vi "TestMatrix.vi"() -> ()   [LabVIEW 2022 SP3]
uses:
  <vilib>/Analysis/2dsp.llb/2D Convolution (DBL).vi
  <vilib>/Analysis/NI_AALPro.lvlib
panel:
  out "Intensity Graph 2":dbl[][](graph)
  out "Power":dbl
  out "Time (s)":dbl
  in  "stop":bool
  out "Intensity Graph":dbl[][](graph)
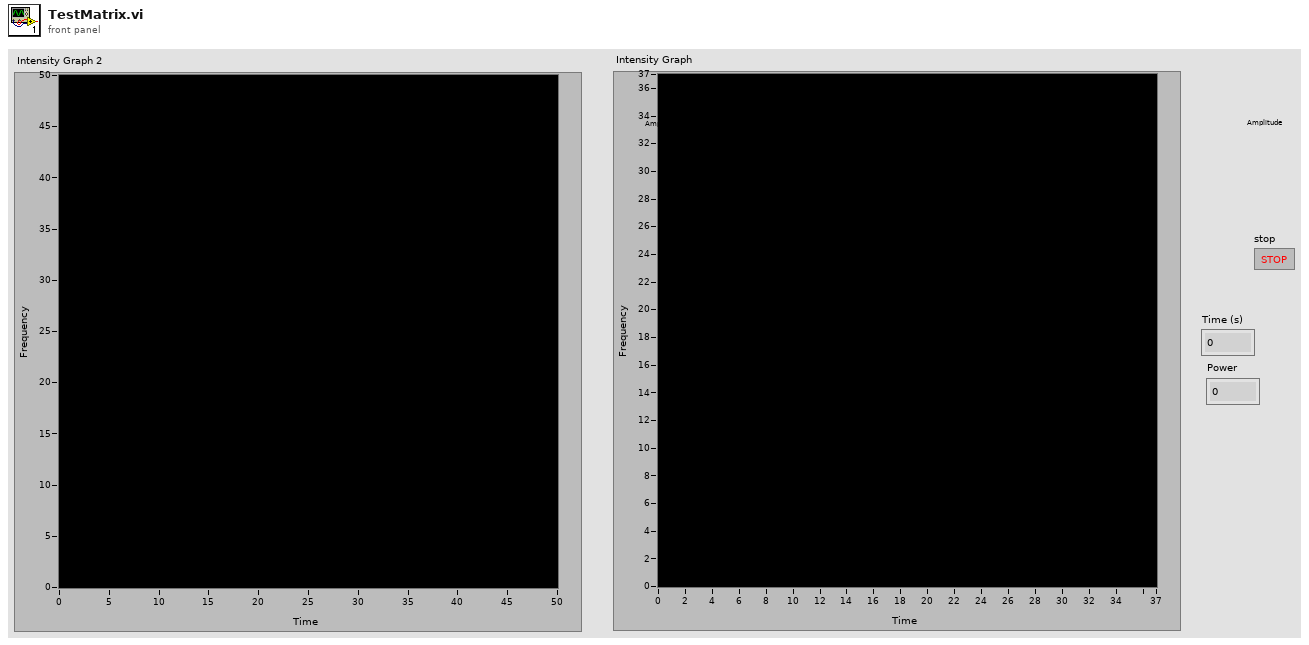
[diagram p1: front panel]
types:
  T1 = enum16{"open", "replace", "create", "open or create", "replace or create", "replace or create with confirmation"}
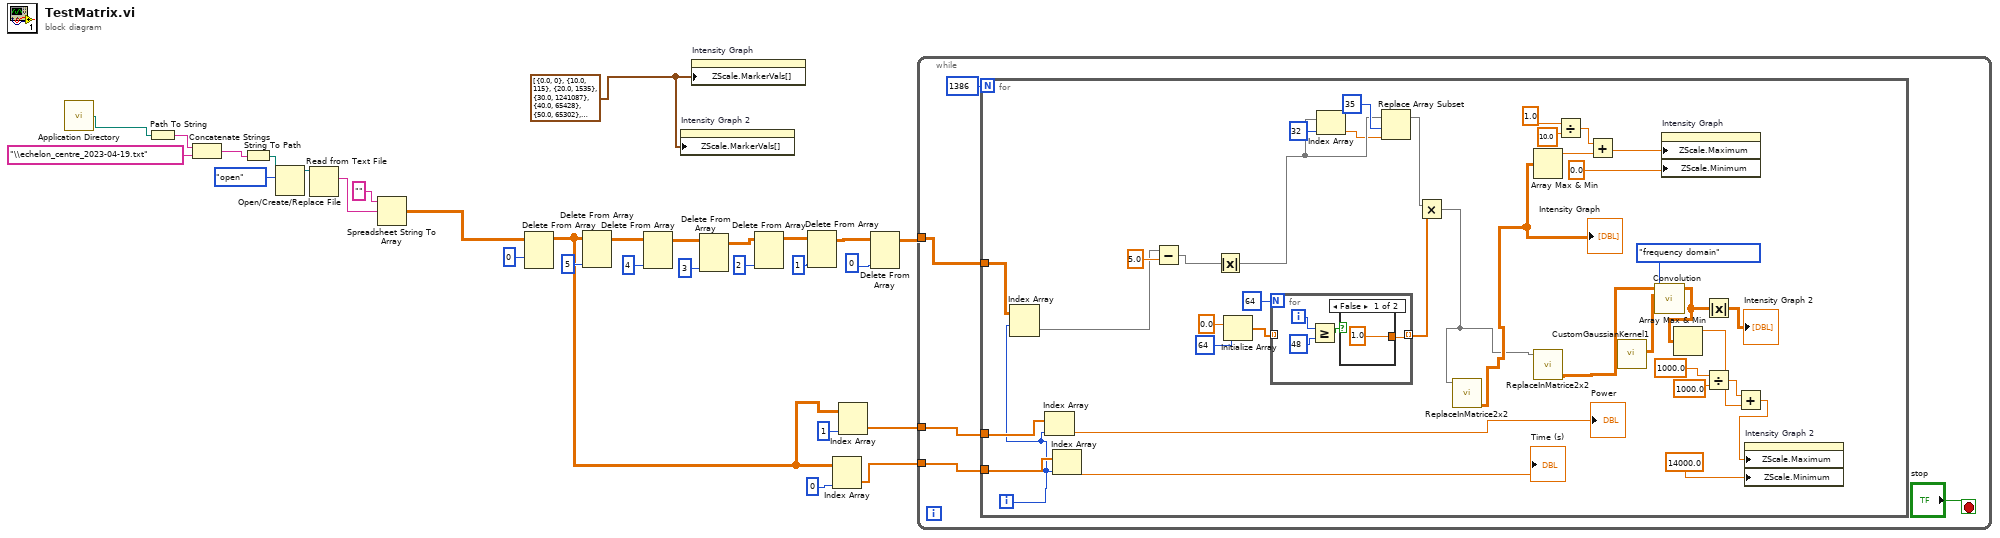
[diagram p0: block diagram]
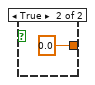
[diagram p2: hidden frame]
diagram:
  w2 = cluster{dbl, u32}[] [{0.0, 0}, {10.0, 115}, {20.0, 1535}, {30.0, 1241087}, {40.0, 65428}, {50.0, 65302}, {60.0, 15925010}, {70.0, 16756736}, {80.0, 16739858}, {90.0, 16712704}, {100.0, 10420224}] ("Z Scale.Marker Values[]")
  n1 = call <vilib>:"Application Directory.vi"() -> ("Application Directory"=w10:path)
  n2 = Path To String(path=w10) -> (string=w29:string)
  n3 = Concatenate Strings(w29, "\\echelon_centre_2023-04-19.txt" ("string")) -> (w27:string)
  n4 = String To Path(string=w27) -> (path=w26:path)
  n5 = Open/Create/Replace File(file path (use dialog)=w26, operation (0:open)=T1."open") -> (refnum out=w24:refnum<file>)  [unwired: 4 in, 2 out]
  n6 = Read from Text File(file (use dialog)=w24) -> (text=w23:string)  [unwired: 3 in, 3 out]
  n7 = Spreadsheet String To Array(format string="", spreadsheet string=w23) -> (array=w11:dbl[][])  [unwired: 2 in]
  n8 = Delete From Array(array=w11, index (row)=0) -> (array with subset deleted=w4:dbl[][])  [unwired: 2 in, 1 out]
  n9 = Delete From Array(array=w4, index (col)=5 ("disabled index (col)")) -> (array with subset deleted=w19:dbl[][])  [unwired: 2 in, 1 out]
  n10 = Delete From Array(array=w19, index (col)=4 ("disabled index (col)")) -> (array with subset deleted=w17:dbl[][])  [unwired: 2 in, 1 out]
  n11 = property on="Intensity Graph 2" class="IntGraph (strict)"("ZScale.MarkerVals[]"=w2) -> ()  [unwired: 2 in, 2 out]
  n12 = property on="Intensity Graph" class="IntGraph (strict)"("ZScale.MarkerVals[]"=w2) -> ()  [unwired: 2 in, 2 out]
  n13 = Delete From Array(array=w17, index (col)=3 ("disabled index (col)")) -> (array with subset deleted=w14:dbl[][])  [unwired: 2 in, 1 out]
  n14 = Delete From Array(array=w14, index (col)=2) -> (array with subset deleted=w13:dbl[][])  [unwired: 2 in, 1 out]
  n15 = Delete From Array(array=w13, index (col)=1 ("disabled index (col)")) -> (array with subset deleted=w8:dbl[][])  [unwired: 2 in, 1 out]
  n16 = Index Array(array=w4, index (col)=0 ("disabled index (col)")) -> (element=w6:dbl[])  [unwired: 1 in]
  n17 = Index Array(array=w4, index (col)=1) -> (element=w3:dbl[])  [unwired: 1 in]
  n18 = Delete From Array(array=w8, index (col)=0) -> (array with subset deleted=w1:dbl[][])  [unwired: 2 in, 1 out]
  n19 = while {
    tunnel: w1 -> [w33]
    tunnel: w6 -> [w32]
    tunnel: w3 -> [w31]
    stop <- "stop" stop-if-true
    n20 = for {
      N: 1386 -> [_]
      tunnel: w33 -> [w68]
      tunnel: w32 -> [w67]
      tunnel: w31 -> [w65]
      i -> [w63]
      n21 = Index Array(array=w68, index (row)=w63) -> (element=w51:dbl[])  [unwired: 1 in]
      n22 = Index Array(array=w65, index=w63) -> (element=→"Power":dbl)
      n23 = Index Array(array=w67, index=w63) -> (element=→"Time (s)":dbl)
      n24 = Subtract(x=w51, y=5.0) -> (x-y=w50:dbl[])
      n25 = Absolute Value(x=w50) -> (abs(x)=w45:dbl[])
      n26 = Initialize Array(0.0 ("element"), 64 ("dimension size")) -> (w39:dbl[])
      n27 = for {
        N: 64 -> [_]
        tunnel: w39 -> [_] mode=indexing
        tunnel: [w73] -> w36 mode=indexing
        i -> [w76]
        n28 = Greater Or Equal?(x=w76, y=48) -> (x >= y?=w74:bool)
        n29 = case shown="False" w74 {
          tunnel: [1.0 0.0] -> w73
          frame False {
          }
          frame True {
          }
        }
      }
      n30 = Index Array(array=w45, index=32) -> (element=w44:dbl)
      n31 = Replace Array Subset(array=w45, new element=w44, index=35) -> (w37:dbl[])
      n32 = Multiply(x=w37, y=w36) -> (x*y=w35:dbl[])
      n33 = call "ReplaceInMatrice2x2.vi"("Input Array"=w35) -> ("Output Array"=w43:dbl[][])  [unwired: 10 in]
      "Intensity Graph" <- w43
      n34 = Array Max & Min(array=w43) -> (max value=w72:dbl)  [unwired: 3 out]
      n35 = call "ReplaceInMatrice2x2.vi"("Input Array"=w35) -> ("Output Array"=w42:dbl[][])  [unwired: 10 in]
      n36 = Divide(x=1.0, y=10.0) -> (x/y=w71:dbl)
      n37 = Add(x=w71, y=w72) -> (x+y=w61:dbl)
      n38 = call "CustomGaussianKernel1.vi"() -> ("array"=w62:dbl[][])  [unwired: 11 in]
      n39 = call-poly <vilib>:"Convolution.vi"("algorithm"=enum32{"direct", "frequency domain"}."frequency domain", "Y"=w62, "X"=w42) -> ("X * Y"=w48:dbl[][])  [unwired: 7 in, 1 out]
      n40 = property on="Intensity Graph" class="IntGraph (strict)"("ZScale.Maximum"=w61, "ZScale.Minimum"=0.0 ("Z Scale.Range:Minimum")) -> ()  [unwired: 2 in, 2 out]
      n41 = Array Max & Min(array=w48) -> (max value=w60:dbl)  [unwired: 3 out]
      n42 = Absolute Value(x=w48) -> (abs(x)=→"Intensity Graph 2":dbl[][])
      n43 = Divide(x=1000.0, y=1000.0) -> (x/y=w59:dbl)
      n44 = Add(x=w59, y=w60) -> (x+y=w56:dbl)
      n45 = property on="Intensity Graph 2" class="IntGraph (strict)"("ZScale.Maximum"=w56, "ZScale.Minimum"=14000.0 ("Z Scale.Range:Minimum")) -> ()  [unwired: 2 in, 2 out]
    }
  }
